vi "Check if robot is connected to the robot (robot).vi"(8 "error in (no error)":errorcluster) -> ()   [LabVIEW 2013]
uses:
  Robot Global Var.vi
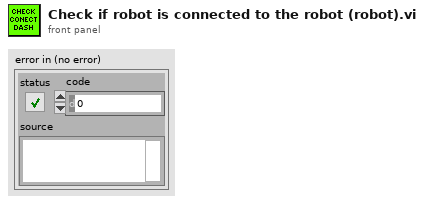
[diagram p1: front panel]
types:
  T1 = cluster{"millisecond timer value":u32, "Slide":i32}
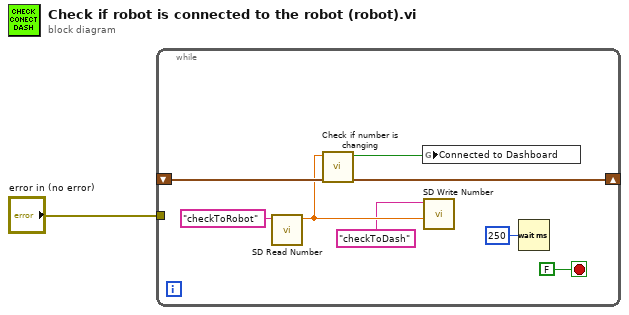
[diagram p0: block diagram]
diagram:
  n1 = while {
    shift-right: [w7] -> _
    shift-left: _ -> [w6]
    tunnel: "error in (no error)" -> [_]
    stop <- FALSE stop-if-true
    n2 = call <vilib>:"SD Read Number.vi"("Name"="checkToRobot") -> ("Numeric"=w3:dbl)  [unwired: 8 in, 2 out]
    n3 = call "Check if number is changing.vi"("Shift in"=w6, "Number to check"=w3) -> ("Shift out"=w7:T1, "Number Changing"=w5:bool)  [unwired: 8 in]
    n4 = global write "Robot Global Var.vi" "Connected to Dashboard"(w5) -> ()
    n5 = call <vilib>:"SD Write Number.vi"("Numeric"=w3, "Name"="checkToDash") -> ()  [unwired: 8 in, 2 out]
    n6 = Wait (ms)(milliseconds to wait=u32 250) -> ()  [unwired: 1 out]
  }
